vi "T2(SubVI).vi"(6 "Sample Rate":dbl, 7 "Write Output to File?":bool=TRUE, 8 "output mode":T1 items=["Standard Function", "Frequency List", "Arbitrary Waveform", "Arbitrary Sequence", "Script"], 9 "Larmor Frequency":dbl=27410000.0 caption="Frequency" format="%.4p", 10 "Pulse Train File":path, 11 "Number of Scans":i32=8) -> (0 "Signal Intensity (Integral)":dbl=0.6544283602926818 format="%0.4f", 1 "T2 Fit":dbl[](graph), 2 "Extracted T2 Decay - Current Scan":waveform(dbl)(graph)={"t0"=timestamp(0 s since 1904-01-01), "dt"=0.0012610340479192938, "Y"=array[3965 elements]} caption="Waveform Graph", 3 "Averaged T2 Decay":waveform(dbl)(graph)={"t0"=timestamp(0 s since 1904-01-01), "dt"=0.0012610340479192938, "Y"=array[3965 elements]} caption="Waveform Graph", 4 "Scan Number":i32=8, 5 "Pulse Echos - Current Scan":waveform(dbl)(graph)={"t0"=timestamp(0 s since 1904-01-01), "dt"=0.0012610340479192938, "Y"=array[3965 elements]} caption="Waveform Graph")   [LabVIEW 2021]
uses:
  <instrlib>/niFgen/niFgen.llb/niFgen Output Mode.ctl
  <instrlib>/niFgen/niFgen.llb/niFgen Waveform Type.ctl
  <instrlib>/niFgen/niFgen.llb/niFgen_ctl Trigger DigEdge - Edge Values (Ring).ctl
  <instrlib>/niFgen/niFgen.llb/niFgen_ctl Trigger Source Values (Ring).ctl
  <instrlib>/niFgen/niFgen.llb/niFgen Trigger Mode.ctl
  <instrlib>/niScope/Controls/niScope acquisition type.ctl
  <instrlib>/niScope/Controls/niScope trigger slope.ctl
  <instrlib>/niScope/Controls/niScope trigger source.ctl
  <vilib>/Analysis/2dsp.llb/Integral Method.ctl
  <vilib>/Analysis/8numeric.llb/1D Numeric Integration.vi
  <vilib>/Utility/file.llb/Read Delimited Spreadsheet (DBL).vi
  <instrlib>/niFgen/niFgen.llb/niFgen Create Waveform (DBL).vi
  <instrlib>/niScope/Configure/Trigger/niScope Configure Trigger Edge.vi
  <instrlib>/niFgen/niFgen.llb/niFgen Configure Digital Edge Start Trigger.vi
  <instrlib>/niScope/Acquire/Fetch/niScope Fetch Cluster.vi
  <vilib>/Waveform/WDTFileIO.llb/Export Waveform To Spreadsheet File.vi
  <vilib>/Analysis/NI_AALPro.lvlib
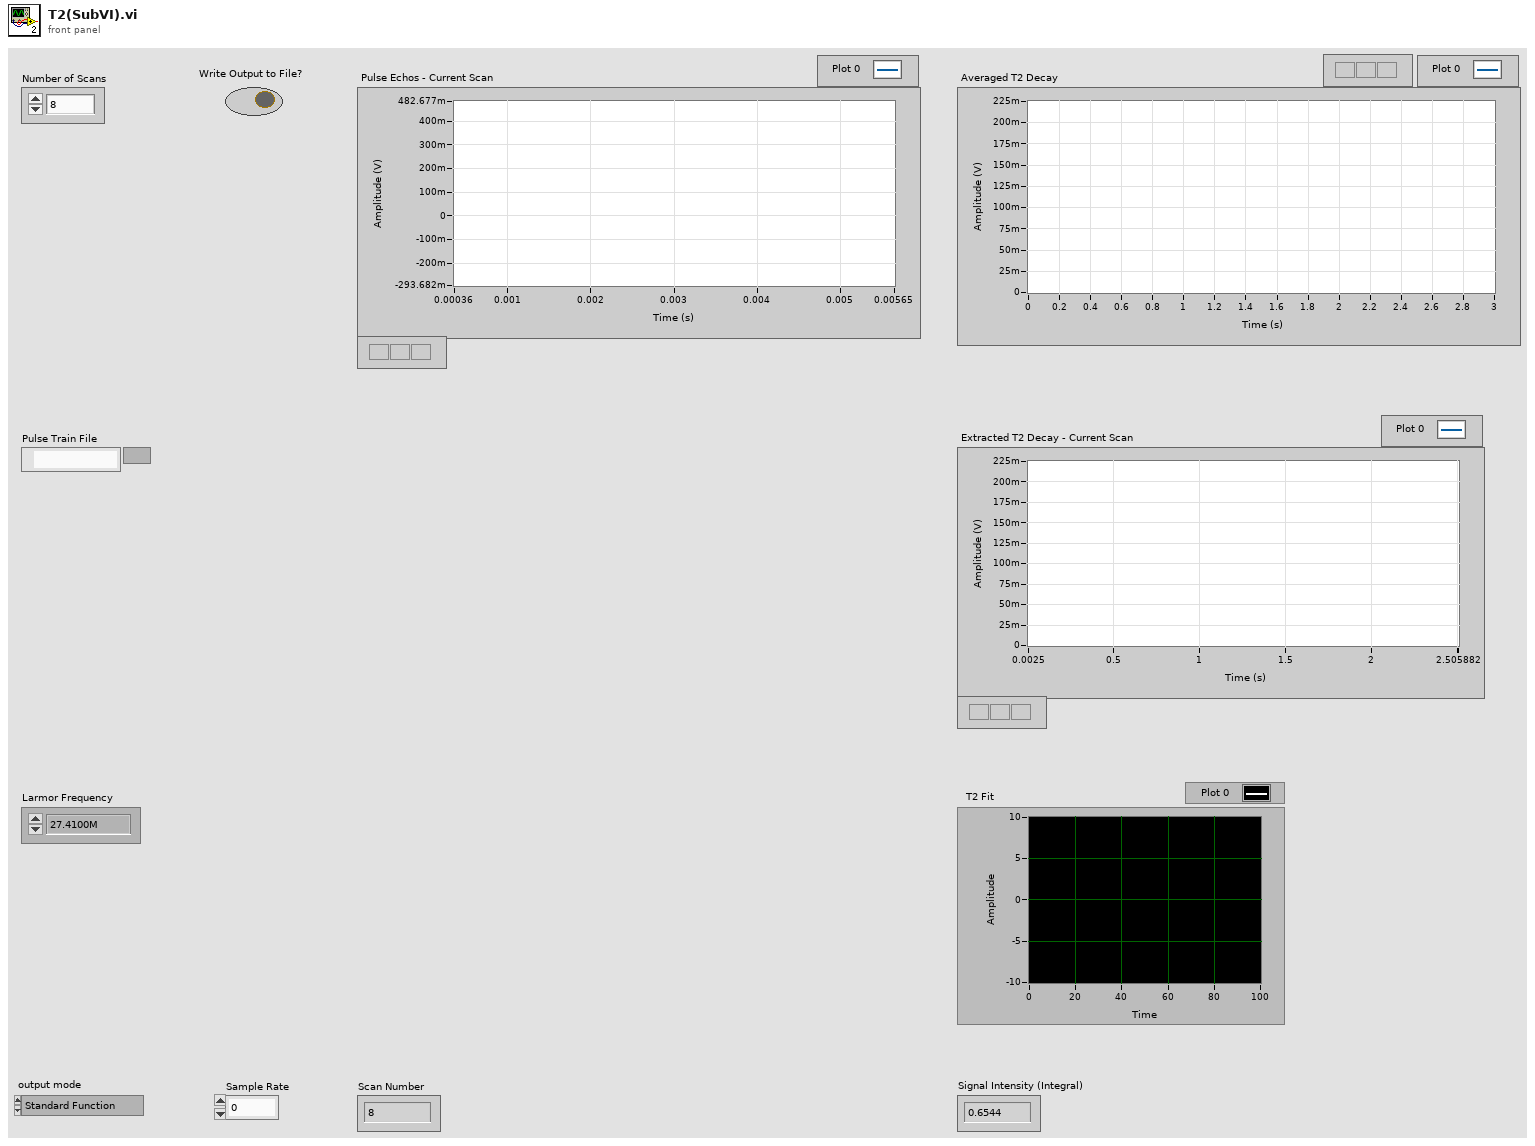
[diagram p1: front panel]
types:
  T1 = typedef "niFgen Output Mode.ctl" = u32
  T2 = typedef "niScope trigger source.ctl" = string
  T3 = typedef "niFgen_ctl Trigger Source Values (Ring).ctl" = string
  T4 = typedef "NI_AALPro.lvlib/Integral Method.ctl" = i32
  T5 = typedef "niScope trigger slope.ctl" = i32
  T6 = typedef "niScope acquisition type.ctl" = i32
  T7 = typedef "niFgen Trigger Mode.ctl" = i32
  T8 = typedef "niFgen_ctl Trigger DigEdge - Edge Values (Ring).ctl" = i32
  T9 = typedef "niFgen Waveform Type.ctl" = i32
  T10 = cluster{"relativeInitialX":dbl, "xIncrement":dbl, "wfm":dbl[]}
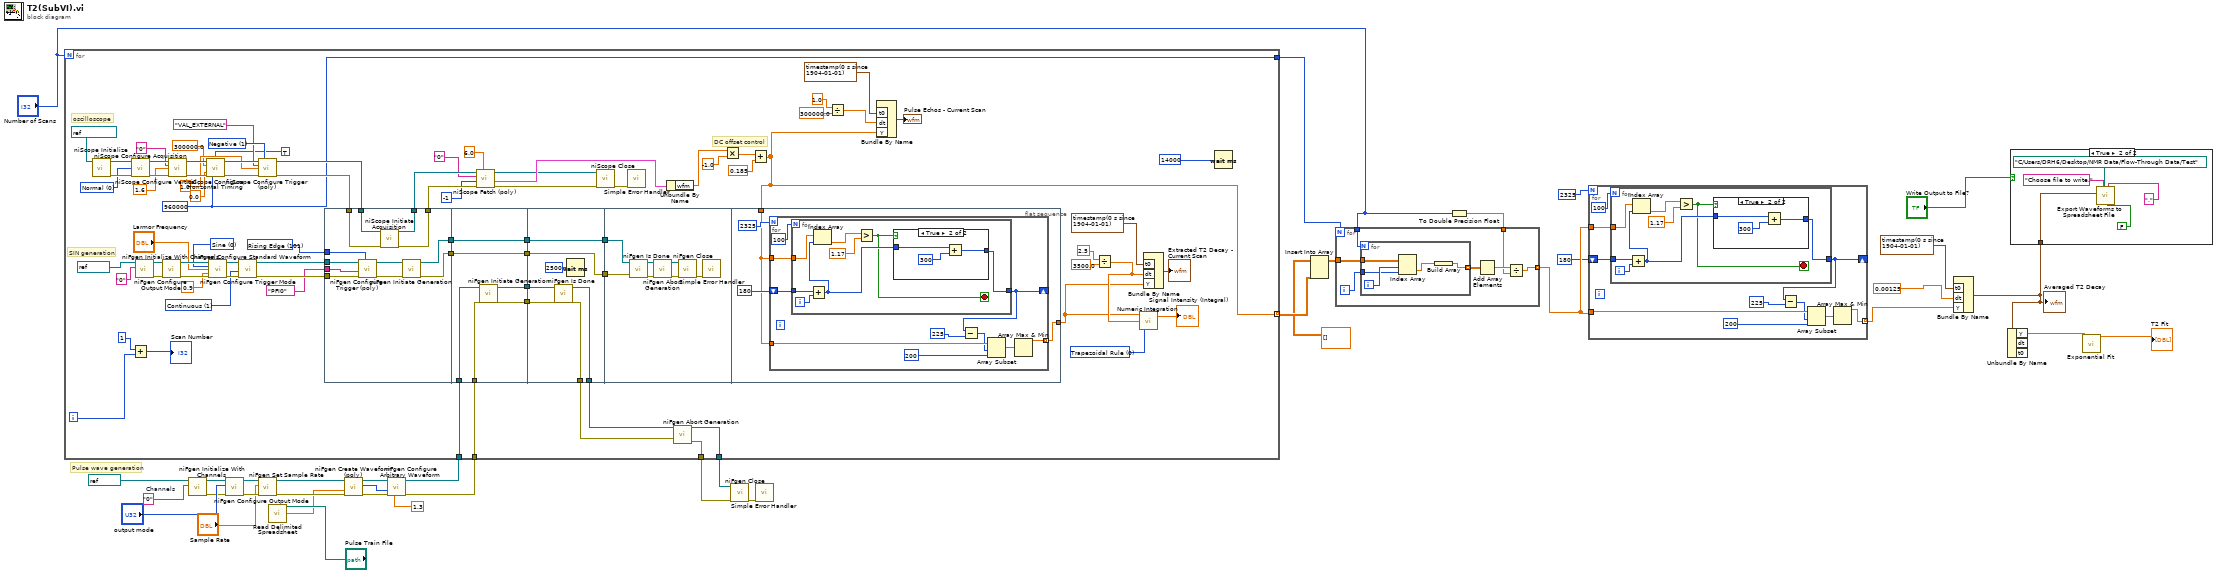
[diagram p0: block diagram]
diagram:
  w15 = "0"  # Channels
  # "Pulse wave generation"
  n1 = call <instrlib>:"niFgen Initialize With Channels.vi"("Channel Name"=w15, "Resource Name"=refnum<k15> "Dev1" ("FGEN Resource Name 2")) -> ("error out"=w12:errorcluster, "Instrument Handle Out"=w11:refnum<k15>)  [unwired: 8 in]
  n2 = call <instrlib>:"niFgen Configure Output Mode.vi"("error in (no error)"=w12, "Output Mode (default: 0=Standard Function)"="output mode", "Instrument Handle"=w11) -> ("error out"=w8:errorcluster, "Instrument Handle Out"=w9:refnum<k15>)  [unwired: 6 in]
  n3 = call <instrlib>:"niFgen Set Sample Rate.vi"("error in (no error)"=w8, "Sample Rate (Samp/s)"="Sample Rate", "Instrument Handle"=w9) -> ("error out"=w5:errorcluster, "Instrument Handle Out"=w6:refnum<k15>)  [unwired: 7 in]
  n4 = call-poly <vilib>:"Read Delimited Spreadsheet.vi"("file path (dialog if empty)"="Pulse Train File") -> ("first row"=w4:dbl[])  [unwired: 9 in, 5 out]
  n5 = call-poly <instrlib>:"niFgen Create Waveform (poly).vi"("error in (no error)"=w5, "Waveform Data Array"=w4, "Instrument Handle"=w6) -> ("error out"=w2:errorcluster, "Waveform Handle"=w1:i32, "Instrument Handle Out"=w3:refnum<k15>)  [unwired: 6 in]
  n6 = call <instrlib>:"niFgen Configure Arbitrary Waveform.vi"("Gain"=1.3, "error in (no error)"=w2, "Waveform Handle"=w1, "Instrument Handle"=w3) -> ("error out"=w17:errorcluster, "Instrument Handle Out"=w18:refnum<k15>)  [unwired: 6 in]
  n7 = for {
    N: "Number of Scans" -> [_]
    tunnel: w17 -> [w101]
    tunnel: w18 -> [w100]
    tunnel: [w99] -> w20
    tunnel: [w98] -> w21
    tunnel: [w38] -> w24 mode=indexing
    tunnel: [w49] -> w27
    i -> [w56]
    w58 = T4 0 items=["Trapezoidal Rule", "Simpson's Rule", "Simpson's 3/8 Rule", "Bode Rule"] ("integration method")
    w49 = 960000 ("min record length")
    w86 = T5 1 items=["Positive", "Negative"] ("trigger slope")
    w87 = T6 0 items=["Normal"=0, "Flex Res"=1, "DDC"=3] ("acquisition Type")
    w106 = T7 1 items=["Single", "Continuous", "Stepped", "Burst"] ("Trigger Mode (default: 1=continuous)")
    w110 = T8 101 items=["Rising Edge"=101, "Falling Edge"=102] ("Edge (Rising)")
    w111 = T9 0 items=["Sine", "Square", "Triangle", "Ramp Up", "Ramp Down", "DC", "Noise", "User"] ("Waveform")
    # "SIN generation"
    # "oscilloscope"
    # "DC offset control"
    n8 = call <instrlib>:"niScope Initialize.vi"("resource name"=refnum<k15> "PXI1Slot6") -> ("instrument handle"=w88:refnum<k15>, "error out"=w89:errorcluster)  [unwired: 13 in]
    n9 = call <instrlib>:"niScope Configure Acquisition.vi"("instrument handle"=w88, "acquisition Type"=w87, "error in"=w89) -> ("instrument handle out"=w91:refnum<k15>, "error out"=w92:errorcluster)  [unwired: 11 in]
    n10 = Add(x=1, y=w56) -> (x+y=→"Scan Number":i32)
    n11 = call <instrlib>:"niFgen Initialize With Channels.vi"("Channel Name"="0", "Resource Name"=refnum<k15> "Dev3" ("Sine Wave Module")) -> ("error out"=w116:errorcluster, "Instrument Handle Out"=w119:refnum<k15>)  [unwired: 8 in]
    n12 = call <instrlib>:"niFgen Configure Output Mode.vi"("error in (no error)"=w116, "Instrument Handle"=w119) -> ("error out"=w115:errorcluster, "Instrument Handle Out"=w118:refnum<k15>)  [unwired: 7 in]
    n13 = call <instrlib>:"niScope Configure Vertical.vi"("instrument handle"=w91, "channels"="0", "vertical range"=1.6, "error in"=w92) -> ("instrument handle out"=w93:refnum<k15>, "error out"=w94:errorcluster)  [unwired: 10 in]
    n14 = call <instrlib>:"niScope Configure Horizontal Timing.vi"("instrument handle"=w93, "enforce realtime"=TRUE, "min sample rate"=300000.0, "reference position"=0.0, "error in"=w94, "min record length"=w49) -> ("instrument handle out"=w95:refnum<k15>, "error out"=w96:errorcluster)  [unwired: 8 in]
    n15 = call <instrlib>:"niFgen Configure Standard Waveform.vi"("Instrument Handle"=w118, "Waveform"=w111, "Frequency"="Larmor Frequency", "Amplitude"=0.9, "error in (no error)"=w115) -> ("Instrument Handle Out"=w117:refnum<k15>, "error out"=w114:errorcluster)  [unwired: 9 in]
    n16 = call <instrlib>:"niFgen Configure Trigger Mode.vi"("error in (no error)"=w114, "Trigger Mode (default: 1=continuous)"=w106, "Instrument Handle"=w117) -> ("error out"=w109:errorcluster, "Instrument Handle Out"=w107:refnum<k15>)  [unwired: 7 in]
    n17 = call-poly <instrlib>:"niScope Configure Trigger (poly).vi"("instrument handle"=w95, "trigger slope"=w86, "trigger source"=T2 "VAL_EXTERNAL", "trigger level"=1.0, "error in"=w96) -> ("instrument handle out"=w80:refnum<k15>, "error out"=w79:errorcluster)  [unwired: 9 in]
    n18 = flat-sequence {
      tunnel: w110 -> [w130]
      tunnel: w109 -> [w129]
      tunnel: T3 "PFI0" ("Source") -> [w128]
      tunnel: w107 -> [w127]
      tunnel: w80 -> [w125]
      tunnel: w79 -> [w124]
      tunnel: [w123] -> w78
      tunnel: [w122] -> w77
      tunnel: [w121] -> w67
      tunnel: [w120] -> w64
      tunnel: w101 -> [w137]
      tunnel: w100 -> [w136]
      tunnel: [w135] -> w71
      tunnel: [w134] -> w70
      tunnel: [w133] -> w68
      tunnel: w67 -> [w133]
      tunnel: [w132] -> w65
      tunnel: w64 -> [w132]
      tunnel: [w143] -> w104
      tunnel: [w142] -> w103
      tunnel: w71 -> [w141]
      tunnel: w70 -> [w140]
      tunnel: [w139] -> w69
      tunnel: w68 -> [w139]
      tunnel: [w138] -> w66
      tunnel: w65 -> [w138]
      tunnel: w69 -> [w146]
      tunnel: w66 -> [w145]
      tunnel: w38 -> [w152]
      tunnel: [w154] -> w48
      frame #0 {
        n19 = call-poly <instrlib>:"niFgen Configure Trigger (poly).vi"("Edge (Rising)"=w130, "error in (no error)"=w129, "Source"=w128, "Instrument Handle"=w127) -> ("error out"=w126:errorcluster, "Instrument Handle Out"=w131:refnum<k15>)  [unwired: 6 in]
        n20 = call <instrlib>:"niScope Initiate Acquisition.vi"("instrument handle"=w125, "error in"=w124) -> ("instrument handle out"=w123:refnum<k15>, "error out"=w122:errorcluster)  [unwired: 12 in]
        n21 = call <instrlib>:"niFgen Initiate Generation.vi"("error in (no error)"=w126, "Instrument Handle"=w131) -> ("error out"=w120:errorcluster, "Instrument Handle Out"=w121:refnum<k15>)  [unwired: 8 in]
      }
      frame #1 {
        n22 = call <instrlib>:"niFgen Initiate Generation.vi"("error in (no error)"=w137, "Instrument Handle"=w136) -> ("error out"=w134:errorcluster, "Instrument Handle Out"=w135:refnum<k15>)  [unwired: 8 in]
      }
      frame #2 {
        n23 = call <instrlib>:"niFgen Is Done.vi"("error in (no error)"=w140, "Instrument Handle"=w141) -> ("error out"=w143:errorcluster, "Instrument Handle Out"=w142:refnum<k15>)  [unwired: 7 in, 1 out]
        n24 = Wait (ms)(milliseconds to wait=u32 2500) -> ()  [unwired: 1 out]
      }
      frame #3 {
        n25 = call <instrlib>:"niFgen Is Done.vi"("error in (no error)"=w145, "Instrument Handle"=w146) -> ("error out"=w149:errorcluster, "Instrument Handle Out"=w148:refnum<k15>)  [unwired: 7 in, 1 out]
        n26 = call <instrlib>:"niFgen Abort Generation.vi"("error in (no error)"=w149, "Instrument Handle"=w148) -> ("error out"=w150:errorcluster, "Instrument Handle Out"=w151:refnum<k15>)  [unwired: 8 in]
        n27 = call <instrlib>:"niFgen Close.vi"("error in (no error)"=w150, "Instrument Handle"=w151) -> ("error out"=w147:errorcluster)  [unwired: 9 in]
        n28 = call <vilib>:"Simple Error Handler.vi"("error in (no error)"=w147) -> ()  [unwired: 4 in, 5 out]
      }
      frame #4 {
        n29 = for {
          N: 2325 -> [_]
          tunnel: [w164] -> w154 mode=indexing
          tunnel: w152 -> [w163]
          shift-right: [w158] -> _
          shift-left: 180 -> [w159]
          tunnel: w152 -> [w157]
          n30 = for {
            N: 100 -> [_]
            tunnel: w157 -> [w169]
            tunnel: w159 -> [w172]
            tunnel: [w167] -> w158
            i -> [w173]
            stop <- w166 stop-if-true
            n31 = Add(x=w172, y=w173) -> (x+y=w168:i32)
            n32 = Index Array(array=w169, index=w168) -> (element=w170:dbl)
            n33 = Greater?(x=w170, y=1.17) -> (0:w166:bool)
            n34 = case shown="True" w166 {
              tunnel: w168 -> [w174 w175]
              tunnel: [w174 w177] -> w167
              frame False {
              }
              frame True {
                n35 = Add(x=w175, y=300) -> (x+y=w177:i32)
              }
            }
          }
          n36 = Subtract(x=w158, y=225) -> (x-y=w160:i32)
          n37 = Array Subset(array=w163, index=w160, length=200 ("y")) -> (w165:dbl[])
          n38 = Array Max & Min(array=w165) -> (max value=w164:dbl)  [unwired: 3 out]
        }
      }
    }
    n39 = call-poly <instrlib>:"niScope Fetch (poly).vi"("timeout"=6.0, "error in"=w77, "numSamples"=-1, "channels"="0", "instrument handle"=w78) -> ("error out"=w50:errorcluster, "waveform"=w53:T10, "instrument handle out"=w51:refnum<k15>)  [unwired: 3 in, 1 out]
    n40 = call <instrlib>:"niScope Close.vi"("instrument handle"=w51, "error in"=w50) -> ("error out"=w97:errorcluster)  [unwired: 13 in]
    n41 = call <vilib>:"Simple Error Handler.vi"("error in (no error)"=w97) -> ()  [unwired: 4 in, 5 out]
    n42 = Unbundle By Name(w53) -> ("wfm"=w42:dbl[])
    n43 = call <instrlib>:"niFgen Abort Generation.vi"("error in (no error)"=w104, "Instrument Handle"=w103) -> ("error out"=w99:errorcluster, "Instrument Handle Out"=w98:refnum<k15>)  [unwired: 8 in]
    n44 = Multiply(x=w42, y=-1.0) -> (x*y=w39:dbl[])
    n45 = Add(x=w39, y=0.185) -> (x+y=w38:dbl[])
    n46 = Divide(x=1.0, y=300000.0) -> (x/y=w43:dbl)
    n47 = Bundle By Name("t0"=timestamp(0 s since 1904-01-01), "dt"=w43, "Y"=w38) -> (→"Pulse Echos - Current Scan":waveform(dbl))  [unwired: 1 in]
    n48 = Divide(x=2.5, y=3500.0) -> (x/y=w59:dbl)
    n49 = call-poly <vilib>:"Numeric Integration.vi"("integration method"=w58, "dt"=w59, "Input Array"=w48) -> ("result"=→"Signal Intensity (Integral)":dbl)  [unwired: 1 out]
    n50 = Bundle By Name("t0"=timestamp(0 s since 1904-01-01), "dt"=w59, "Y"=w48) -> (→"Extracted T2 Decay - Current Scan":waveform(dbl))  [unwired: 1 in]
    n51 = Wait (ms)(milliseconds to wait=u32 14000 ("Delay Time (ms)")) -> ()  [unwired: 1 out]
  }
  n52 = call <instrlib>:"niFgen Close.vi"("error in (no error)"=w20, "Instrument Handle"=w21) -> ("error out"=w19:errorcluster)  [unwired: 9 in]
  n53 = call <vilib>:"Simple Error Handler.vi"("error in (no error)"=w19) -> ()  [unwired: 4 in, 5 out]
  n54 = Insert Into Array(array=dbl[][] [], new element=w24) -> (w22:dbl[][])  [unwired: 2 in]
  n55 = To Double Precision Float(number="Number of Scans") -> (double precision float=w25:dbl)
  n56 = for {
    N: w27 -> [_]
    tunnel: w22 -> [w184]
    tunnel: [w180] -> w31 mode=indexing
    tunnel: "Number of Scans" -> [w179]
    tunnel: w25 -> [w178]
    i -> [w183]
    n57 = for {
      N: w179 -> [_]
      tunnel: w184 -> [w189]
      tunnel: w183 -> [w187]
      tunnel: [w185] -> w182 mode=indexing
      i -> [w188]
      n58 = Index Array(array=w189, index (row)=w188, index (col)=w187) -> (element=w186:dbl)
      n59 = Build Array(w186) -> (w185:dbl[])
    }
    n60 = Add Array Elements(numeric array=w182) -> (sum=w181:dbl)
    n61 = Divide(x=w181, y=w178) -> (x/y=w180:dbl)
  }
  n62 = for {
    N: 2325 -> [_]
    tunnel: [w198] -> w34 mode=indexing
    tunnel: w31 -> [w197]
    shift-right: [w192] -> _
    shift-left: 180 -> [w193]
    tunnel: w31 -> [w191]
    n63 = for {
      N: 100 -> [_]
      tunnel: w191 -> [w203]
      tunnel: w193 -> [w206]
      tunnel: [w201] -> w192
      i -> [w207]
      stop <- w200 stop-if-true
      n64 = Add(x=w206, y=w207) -> (x+y=w202:i32)
      n65 = Index Array(array=w203, index=w202) -> (element=w204:dbl)
      n66 = Greater?(x=w204, y=1.17) -> (0:w200:bool)
      n67 = case shown="True" w200 {
        tunnel: w202 -> [w208 w209]
        tunnel: [w208 w211] -> w201
        frame False {
        }
        frame True {
          n68 = Add(x=w209, y=300) -> (x+y=w211:i32)
        }
      }
    }
    n69 = Subtract(x=w192, y=225) -> (x-y=w194:i32)
    n70 = Array Subset(array=w197, index=w194, length=200 ("y")) -> (w199:dbl[])
    n71 = Array Max & Min(array=w199) -> (max value=w198:dbl)  [unwired: 3 out]
  }
  n72 = Bundle By Name("t0"=timestamp(0 s since 1904-01-01), "dt"=0.00125 ("y"), "Y"=w34) -> (w36:waveform(dbl))  [unwired: 1 in]
  "Averaged T2 Decay" <- w36
  n73 = Unbundle By Name(w36) -> ("Y"=w35:dbl[])  [unwired: 2 out]
  n74 = case shown="True" "Write Output to File?" {
    tunnel: w36 -> [_ w214]
    frame False {
    }
    frame True {
      n75 = call-poly <vilib>:"Export Waveforms to Spreadsheet File.vi"("header? (write header:T)"=FALSE, "delimiter (Tab)"=",", "prompt"="Choose file to write.", "waveform"=w214, "file path (dialog if empty)"=path "C:/Users/DRH6/Desktop/NMR Data/Flow-Through Data/Test") -> ()  [unwired: 5 in, 2 out]
    }
  }
  n76 = call <vilib>:"Exponential Fit.vi"("Y"=w35) -> ("Best Exponential Fit"=→"T2 Fit":dbl[])  [unwired: 9 in, 5 out]
